vi "test_server.vi"() -> ()   [LabVIEW 2017, in "server.lvlib"]
doc: "This template is for the Queued Message Handler design pattern.\n\nThe Event Handling Loop generates messages based on user interface actions.\n\nThe Message Handling Loop processes messages generated by the Event Handling Loop, or by other messages. The messages are string values, so new messages can be added easily to the Message Cases case structure in the Message Handling Loop. Each message cluster can also provide an optional value for Message Data, which is a variant that can be converted to whatever message-specific data is required."
uses:
  controls/UI Data.ctl
  support/Message Queue/Enqueue Message (Single).vi
  <vilib>/Utility/error.llb/Error Cluster From Error Code.vi
  <vilib>/ErrorRing/Error Ring.xnode
  server.lvlib
  support/Message Queue/Message Queue.lvlib
  support/User Event - Stop/User Event - Stop.lvlib
  logger/logger.lvlib
panel:
  out "Status":string
  in  "Exit":bool
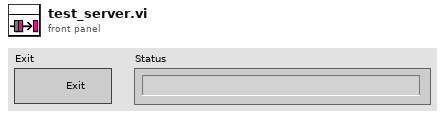
[diagram p1: front panel]
types:
  T1 = typedef "UI Data.ctl" = cluster{"Boolean":bool, "String":string, "Numeric":dbl, "Data Display Ref":refnum<vi>, "Exit Button Ref":refnum<vi>}
  T2 = typedef "Message Queue.lvlib/All Message Queues.ctl" = cluster{"MHL":refnum<queue>, "Server":refnum<queue>, "DataProcessing":refnum<queue>, "Worker":refnum<queue>}
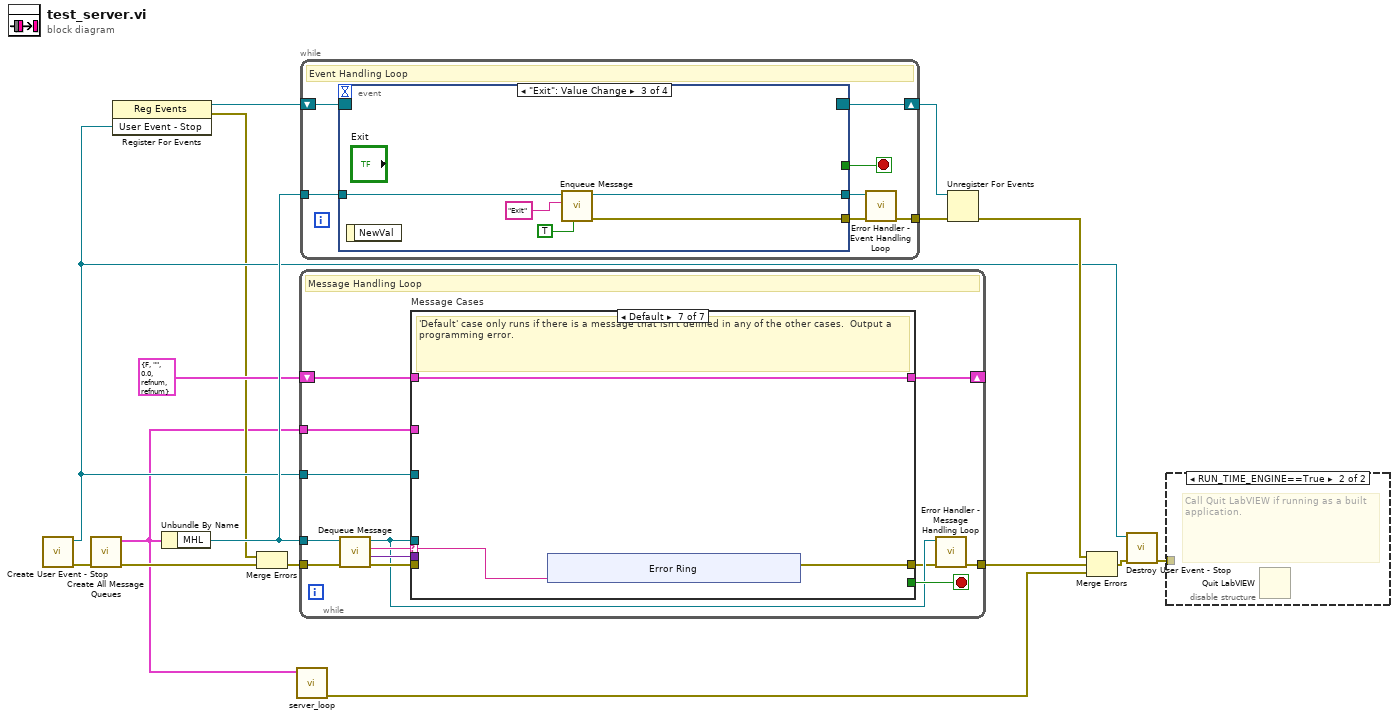
[diagram p0: block diagram]
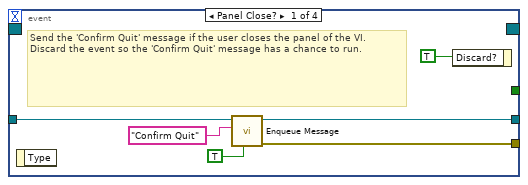
[diagram p3: hidden frame]
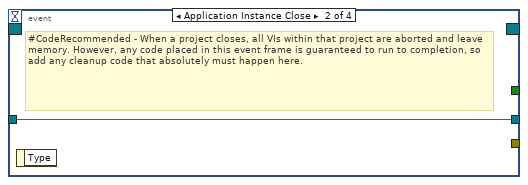
[diagram p4: hidden frame]
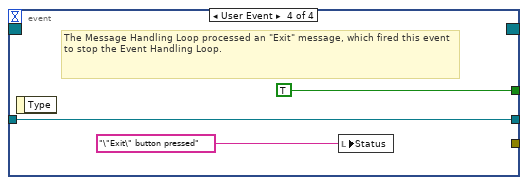
[diagram p5: hidden frame]
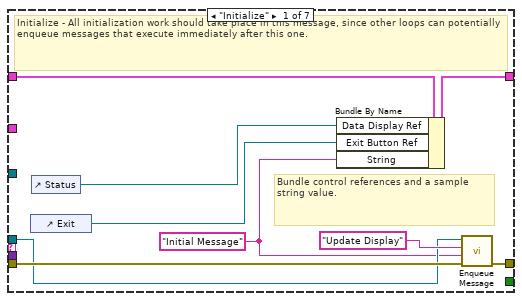
[diagram p6: hidden frame]
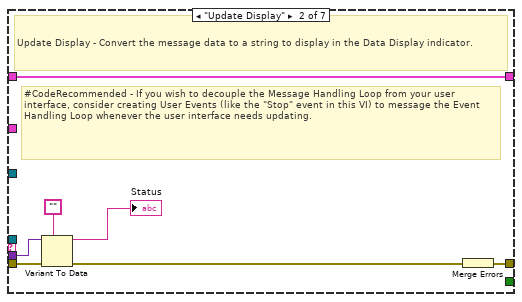
[diagram p7: hidden frame]
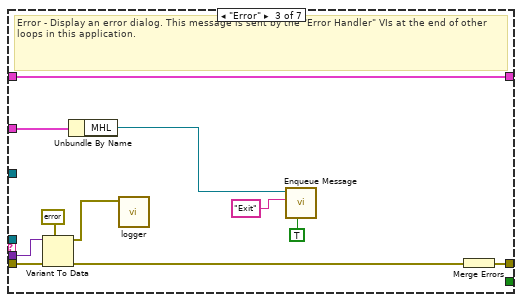
[diagram p8: hidden frame]
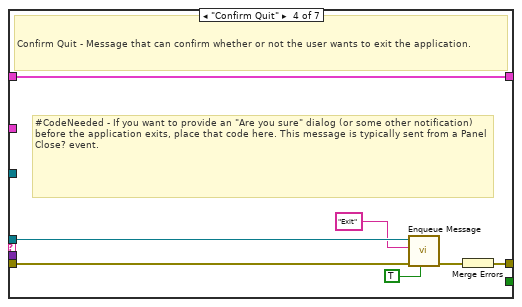
[diagram p9: hidden frame]
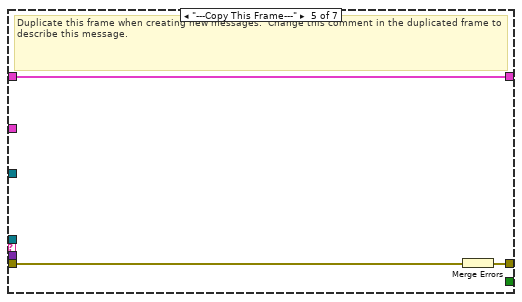
[diagram p10: hidden frame]
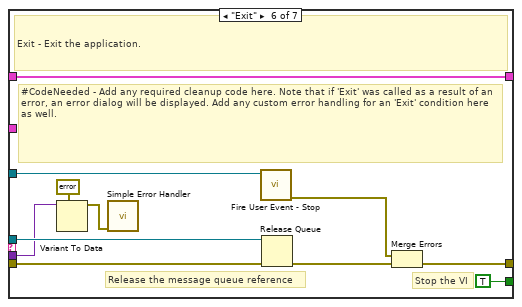
[diagram p11: hidden frame]
diagram:
  n1 = call "Create User Event - Stop.vi"() -> ("error out"=w13:errorcluster, "User Event - Stop"=w5:refnum<user-event>)  [unwired: 10 in]
  n2 = call "Create All Message Queues.vi"("error in (no error)"=w13) -> ("error out"=w16:errorcluster, "Message Queues out"=w2:T2)  [unwired: 9 in]
  n3 = register-events(w5) -> (reference out=w6:refnum<event-registration>, error out=w3:errorcluster)  [unwired: 2 in]
  n4 = Unbundle By Name(w2) -> ("MHL"=w14:refnum<queue>)
  n5 = Merge Errors(w3, w16) -> (w4:errorcluster)
  n6 = call "server_loop.vi"("Message Queues"=w2) -> ("error out"=w1:errorcluster)  [unwired: 10 in]
  n7 = while {
    tunnel: w14 -> [w21]
    shift-right: [w28] -> _
    shift-left: T1 {"Boolean"=FALSE, "String"="", "Numeric"=0.0, "Data Display Ref"=refnum, "Exit Button Ref"=refnum} ("Data Cluster") -> [w29]
    tunnel: w5 -> [w26]
    tunnel: w4 -> [w25]
    tunnel: [w19] -> w15
    tunnel: w2 -> [w17]
    stop <- w27 stop-if-true
    # "Message Handling Loop"
    n8 = call "Dequeue Message.vi"("error in (no error)"=w25, "Message Queue"=w21) -> ("error out"=w24:errorcluster, "Message Data"=w22:variant, "Message"=w23:string, "dup Message Queue"=w20:refnum<queue>)  [unwired: 6 in]
    n9 = case "Message Cases" shown="Default" w23 {
      selector: w23 -> [_ _ _ _ _ _ w78]
      tunnel: w20 -> [w31 _ _ w59 _ w77 _]
      tunnel: w24 -> [w37 w43 w56 w63 w66 w70 _]
      tunnel: [w38 w44 w52 w61 w64 w73 w79] -> w18
      tunnel: w29 -> [w36 w45 w55 w62 w65 w76 w80]
      tunnel: [w35 w45 w55 w62 w65 w76 w80] -> w28
      tunnel: [_ _ _ _ _ TRUE _] -> w27
      tunnel: w22 -> [_ w42 w54 _ _ w67 _]
      tunnel: w26 -> [_ _ _ _ _ w72 _]
      tunnel: w17 -> [_ _ w47 _ _ _ _]
      frame "Initialize" {
        w30 = "Initial Message" ("Initial Message")
        # "Bundle control references and a sample string value."
        # "Initialize - All initialization work should take place in this message, since other loops can potentially enqueue messages that execute immediately after this one."
        n10 = control-ref of="Exit"() -> (w33:refnum<vi>)
        n11 = control-ref of="Status"() -> (w34:refnum<vi>)
        n12 = Bundle By Name(cluster=w36, "Data Display Ref"=w34, "Exit Button Ref"=w33, "String"=w30) -> (w35:T1)
        n13 = call-poly "Enqueue Message.vi"("error in (no error)"=w37, "Message Data"=w30, "Message"="Update Display", "Message Queue"=w31) -> ("error out"=w38:errorcluster)  [unwired: 6 in, 1 out]
      }
      frame "Update Display" {
        # "#CodeRecommended - If you wish to decouple the Message Handling Loop from your user interface, consider creating User Events (like the \"Stop\" event in this VI) to message the Event Handling Loop whenever the user interface needs updating."
        # "Update Display - Convert the message data to a string to display in the Data Display indicator."
        n14 = Variant To Data(error in=w43, type="", Variant=w42) -> (data=→"Status":string, error out=w40:errorcluster)
        n15 = Merge Errors(w40) -> (w44:errorcluster)
      }
      frame "Error" {
        # "Error - Display an error dialog. This message is sent by the \"Error Handler\" VIs at the end of other loops in this application."
        n16 = Variant To Data(error in=w56, type=errorcluster {"status"=FALSE, "code"=0, "source"=""} ("error constant"), Variant=w54) -> (data=w51:errorcluster, error out=w50:errorcluster)
        n17 = Unbundle By Name(w47) -> ("MHL"=w46:refnum<queue>)
        n18 = call "logger.vi"("error in (no error)"=w51) -> ()  [unwired: 11 in]
        n19 = call-poly "Enqueue Message.vi"("Priority Message? (F)"=TRUE, "Message"="Exit", "Message Queue"=w46) -> ()  [unwired: 7 in, 2 out]
        n20 = Merge Errors(w50) -> (w52:errorcluster)
      }
      frame "Confirm Quit" {
        # "#CodeNeeded - If you want to provide an \"Are you sure\" dialog (or some other notification) before the application exits, place that code here. This message is typically sent from a Panel Close? event."
        # "Confirm Quit - Message that can confirm whether or not the user wants to exit the application."
        n21 = call-poly "Enqueue Message.vi"("Priority Message? (F)"=TRUE, "error in (no error)"=w63, "Message"="Exit", "Message Queue"=w59) -> ("error out"=w60:errorcluster)  [unwired: 6 in, 1 out]
        n22 = Merge Errors(w60) -> (w61:errorcluster)
      }
      frame "---Copy This Frame---" {
        # "Duplicate this frame when creating new messages.  Change this comment in the duplicated frame to describe this message."
        n23 = Merge Errors(w66) -> (w64:errorcluster)
      }
      frame "Exit" {
        # "Stop the VI"
        # "Release the message queue reference"
        # "#CodeNeeded - Add any required cleanup code here. Note that if 'Exit' was called as a result of an error, an error dialog will be displayed. Add any custom error handling for an 'Exit' condition here as well."
        # "Exit - Exit the application."
        n24 = Variant To Data(type=errorcluster {"status"=FALSE, "code"=0, "source"=""} ("error constant"), Variant=w67) -> (data=w68:errorcluster)  [unwired: 1 in, 1 out]
        n25 = call <vilib>:"Simple Error Handler.vi"("error in (no error)"=w68) -> ()  [unwired: 4 in, 5 out]
        n26 = call "Fire User Event - Stop.vi"("User Event - Stop"=w72) -> ("error out"=w71:errorcluster)  [unwired: 10 in]
        n27 = Release Queue(queue=w77, error in (no error)=w70) -> (error out=w74:errorcluster)  [unwired: 1 in, 2 out]
        n28 = Merge Errors(w71, w74) -> (w73:errorcluster)
      }
      frame Default {
        # "'Default' case only runs if there is a message that isn't defined in any of the other cases.  Output a programming error."
        n29 = xnode "Error Ring"("parameter 0"=w78) -> ("error out"=w79:errorcluster)
      }
    }
    n30 = call "Error Handler - Message Handling Loop.vi"("error in (no error)"=w18, "Message Queue"=w20) -> ("dup error in"=w19:errorcluster)  [unwired: 8 in, 1 out]
  }
  n31 = while {
    tunnel: w14 -> [w94]
    shift-right: [w92] -> w10
    shift-left: w6 -> [w93]
    tunnel: [w88] -> w7
    stop <- w90 stop-if-true
    # "Event Handling Loop"
    n32 = event shown="[2] \"Exit\": Value Change" {
      selector: w93 -> [_ _ _ _]
      dyn-events: [_ _ _ _] -> w92
      timeout: _ -> [_ _ _ _]
      tunnel: [_ _ _ TRUE ("Discard?")] -> w90
      tunnel: w94 -> [w99 w101 w106 w109]
      tunnel: [w98 _ w105 _] -> w91
      tunnel: [w97 w101 w104 w109] -> w89
      event Panel Close? {
        # "Send the 'Confirm Quit' message if the user closes the panel of the VI. Discard the event so the 'Confirm Quit' message has a chance to run."
        n33 = event-data() -> ()  [unwired: 1 in, 1 out]
        n34 = call-poly "Enqueue Message.vi"("Priority Message? (F)"=TRUE, "Message"="Confirm Quit", "Message Queue"=w99) -> ("error out"=w98:errorcluster, "dup Message Queue"=w97:refnum<queue>)  [unwired: 7 in]
        n35 = event-data("Discard?"=TRUE) -> ()  [unwired: 1 in, 1 out]
      }
      event Application Instance Close {
        # "#CodeRecommended - When a project closes, all VIs within that project are aborted and leave memory. However, any code placed in this event frame is guaranteed to run to completion, so add any cleanup code that absolutely must happen here."
        n36 = event-data() -> ()  [unwired: 1 in, 1 out]
      }
      event "Exit": Value Change {
        n37 = event-data() -> ()  [unwired: 1 in, 1 out]
        n38 = call-poly "Enqueue Message.vi"("Priority Message? (F)"=TRUE, "Message"="Exit", "Message Queue"=w106) -> ("error out"=w105:errorcluster, "dup Message Queue"=w104:refnum<queue>)  [unwired: 7 in]
      }
      event User Event {
        # "The Message Handling Loop processed an \"Exit\" message, which fired this event to stop the Event Handling Loop."
        n39 = event-data() -> ()  [unwired: 1 in, 1 out]
        n40 = local write "Status"("\"Exit\" button pressed" ("VI Stopped")) -> ()
      }
    }
    n41 = call "Error Handler - Event Handling Loop.vi"("error in (no error)"=w91, "Message Queue"=w89) -> ("dup error in"=w88:errorcluster)  [unwired: 8 in, 1 out]
  }
  n42 = Unregister For Events(event registration refnum=w10, error in=w7) -> (error out=w11:errorcluster)
  n43 = Merge Errors(w11, w15, w1) -> (w12:errorcluster)
  n44 = call "Destroy User Event - Stop.vi"("error in (no error)"=w12, "User Event - Stop"=w5) -> ("error out"=w8:errorcluster)  [unwired: 9 in]
  n45 = disable-structure shown="RUN_TIME_ENGINE==True" {
    disable-tunnel: w8 -> [_ _]
    frame condition #0 (active) {
    }
    frame condition #1 {
      # "Call Quit LabVIEW if running as a built application."
      n46 = Quit LabVIEW() -> ()  [unwired: 1 in]
    }
  }
